vi "create new PID.vi"(11 "PID in":T1={"ID"="", "Setpoint"=refnum, "Process Variable"=refnum, "Output"=refnum, "PID gains"={"proportional gain (Kc)"=1.0, "integral time (Ti, min)"=0.01, "derivative time (Td, min)"=0.0}, "output range"={"output high"=100.0, "output low"=-100.0}} {"output range"."output low" format="%.2f"; "output range"."output high" format="%.2f"}) -> (3 "PID out":T1={"ID"="", "Setpoint"=refnum, "Process Variable"=refnum, "Output"=refnum, "PID gains"={"proportional gain (Kc)"=1.0, "integral time (Ti, min)"=0.01, "derivative time (Td, min)"=0.0}, "output range"={"output high"=100.0, "output low"=-100.0}} {"output range"."output low" format="%.2f"; "output range"."output high" format="%.2f"})   [LabVIEW 2014]
doc: "Creates a new PID Loop configuration with properly named Channel Objects for the Setpoint, Process Variable, and Output parameters."
uses:
  <vilib>/NI/Tag Bus Module Framework/channel/TBM channel.lvclass
  <vilib>/NI/Tag Bus Module Framework/channel/channel classification.ctl
  <vilib>/NI/Tag Bus/tag/Data Type.ctl
  <vilib>/NI/Tag Bus/tag/tag descriptor.lvclass
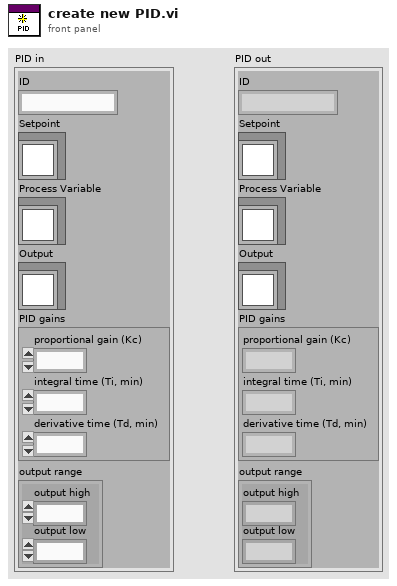
[diagram p1: front panel]
types:
  T1 = cluster{"ID":string, "Setpoint":refnum<class "TBM channel.lvclass">, "Process Variable":refnum<class "TBM channel.lvclass">, "Output":refnum<class "TBM channel.lvclass">, "PID gains":cluster{"proportional gain (Kc)":dbl, "integral time (Ti, min)":dbl, "derivative time (Td, min)":dbl}, "output range":cluster{"output high":dbl, "output low":dbl}}
  T2 = typedef "TBM channel.lvclass/channel classification.ctl" = enum16{"input data", "output data", "processing parameter", "processing result"}
  T3 = typedef "tag bus.lvlib/tag descriptor.lvclass/Data Type.ctl" = enum16{"Double", "Single", "I64", "I32", "I16", "I8", "U64", "U32", "U16", "U8", "Boolean", "String", "Array of Double", "Array of Single", "Array of I64", "Array of I32", "Array of I16", "Array of I8", "Array of U64", "Array of U32", "Array of U16", "Array of U8", "Array of Boolean", "Array of String"}
  T4 = cluster{"proportional gain (Kc)":dbl, "integral time (Ti, min)":dbl, "derivative time (Td, min)":dbl}
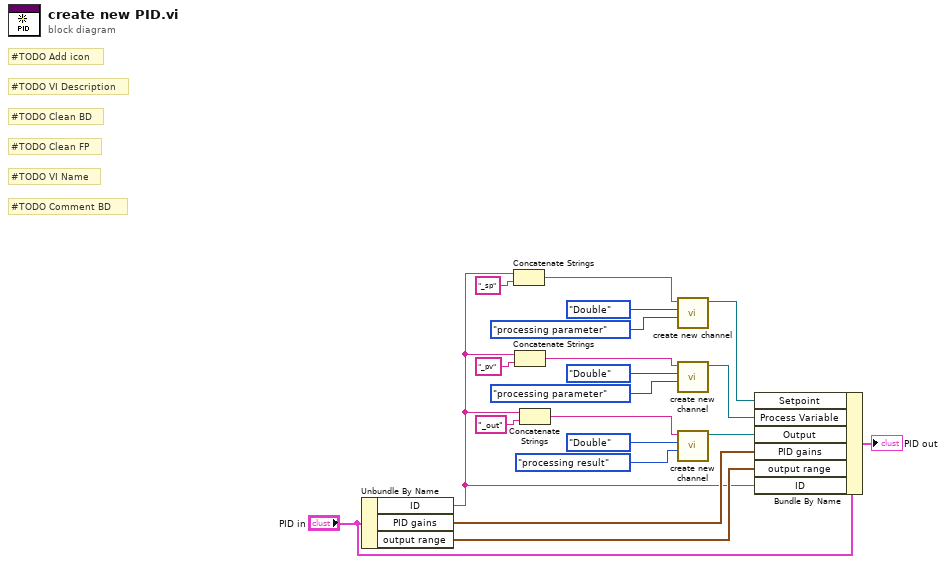
[diagram p0: block diagram]
diagram:
  # "#TODO Comment BD"
  # "#TODO VI Name"
  # "#TODO Clean FP"
  # "#TODO Clean BD"
  # "#TODO VI Description"
  # "#TODO Add icon"
  n1 = Unbundle By Name("PID in") -> ("ID"=w2:string, "PID gains"=w4:T4, "output range"=w3:cluster{"output high":dbl, "output low":dbl})
  n2 = Concatenate Strings(w2, "_sp") -> (w7:string)
  n3 = Concatenate Strings(w2, "_pv") -> (w13:string)
  n4 = Concatenate Strings(w2, "_out") -> (w14:string)
  n5 = call <vilib>:"create new channel.vi"("channel classification"=channel_classification."processing parameter", "data type"=Data_Type."Double", "channel name"=w7) -> ("channel"=w20:refnum<class "TBM channel.lvclass">)  [unwired: 8 in]
  n6 = call <vilib>:"create new channel.vi"("channel classification"=channel_classification."processing parameter", "data type"=Data_Type."Double", "channel name"=w13) -> ("channel"=w19:refnum<class "TBM channel.lvclass">)  [unwired: 8 in]
  n7 = call <vilib>:"create new channel.vi"("channel classification"=channel_classification."processing result", "data type"=Data_Type."Double", "channel name"=w14) -> ("channel"=w18:refnum<class "TBM channel.lvclass">)  [unwired: 8 in]
  n8 = Bundle By Name(cluster="PID in", "Setpoint"=w20, "Process Variable"=w19, "Output"=w18, "PID gains"=w4, "output range"=w3, "ID"=w2) -> (→"PID out":T1)
